vi "Coerce_Timing.vi"(11 "Timing_In":T1 {"Frequency(Hz)" min=10000.0 max=25000000.0 step=100.0 format="%#_6p"; "T_HD_DAT(ns)" step=1.0 format="%#_5g"; "T_SU_STA(ns)" min=0.0 step=1.0 format="%#_5g"; "T_HD_STA(ns)" min=0.0 step=1.0 format="%#_5g"; "T_SU_STO(ns)" min=0.0 step=1.0 format="%#_5g"; "T_BUF(ns)" min=0.0 step=1.0 format="%#_5g"; "T_HIGH(ns)" min=0.0 step=1.0 format="%#_5g"; "T_LOW(ns)" min=0.0 step=1.0 format="%#_5g"; "T_SU_DAT(ns)" step=1.0 format="%#_5g"}) -> (3 "Timing_Out":T1 {"Frequency(Hz)" min=10000.0 max=25000000.0 step=100.0 format="%#_6p"; "T_HD_DAT(ns)" step=1.0 format="%#_5g"; "T_SU_STA(ns)" min=0.0 step=1.0 format="%#_5g"; "T_HD_STA(ns)" min=0.0 step=1.0 format="%#_5g"; "T_SU_STO(ns)" min=0.0 step=1.0 format="%#_5g"; "T_BUF(ns)" min=0.0 step=1.0 format="%#_5g"; "T_HIGH(ns)" min=0.0 step=1.0 format="%#_5g"; "T_LOW(ns)" min=0.0 step=1.0 format="%#_5g"; "T_SU_DAT(ns)" step=1.0 format="%#_5g"})   [LabVIEW 2021, in "Unary.lvlib"]
uses:
  Unary.lvlib
  TypeDef/I2C_Bus_Timing.ctl
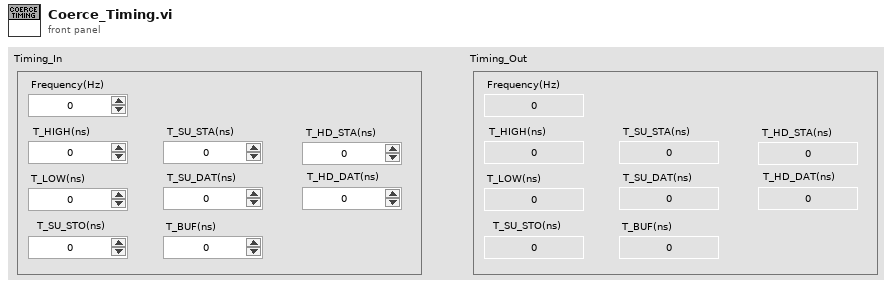
[diagram p1: front panel]
types:
  T1 = typedef "Unary.lvlib/I2C_Bus_Timing.ctl" = cluster{"Frequency(Hz)":dbl, "T_HIGH(ns)":dbl, "T_LOW(ns)":dbl, "T_SU_STO(ns)":dbl, "T_SU_STA(ns)":dbl, "T_SU_DAT(ns)":dbl, "T_BUF(ns)":dbl, "T_HD_STA(ns)":dbl, "T_HD_DAT(ns)":dbl}
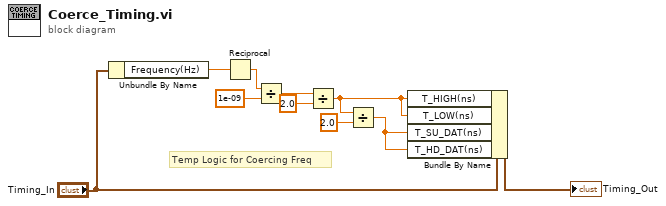
[diagram p0: block diagram]
diagram:
  # "Temp Logic for Coercing Freq"
  n1 = Unbundle By Name("Timing_In") -> ("Frequency(Hz)"=w8:dbl)
  n2 = Reciprocal(x=w8) -> (1/x=w7:dbl)
  n3 = Divide(x=w7, y=1e-09) -> (x/y=w5:dbl)
  n4 = Divide(x=w5, y=2.0) -> (x/y=w1:dbl)
  n5 = Divide(x=w1, y=2.0) -> (x/y=w2:dbl)
  n6 = Bundle By Name(cluster="Timing_In", "T_HIGH(ns)"=w1, "T_LOW(ns)"=w1, "T_SU_DAT(ns)"=w2, "T_HD_DAT(ns)"=w2) -> (→"Timing_Out":T1)
